vi "StateNoteHandling.vi"(0 "Master State In":T1(ring)) -> ()   [LabVIEW 2023]
doc: "This VI performs all of the calculations and decisions related to the swerve drive."
uses:
  <vilib>/Rock Robotics/WPI/ThirdParty/REV Robotics/REVLib/Typedef/Spark MAX Limit Switch Polarity.ctl
  5f0eb4dc-af05-48a2-bc5f-2393b2339903.vi
  GlobalDriverStationCommands.vi
  GlobalElevator.vi
  GlobalNoteHandling.vi
  GlobalPoseAndTargeting.vi
  GlobalShooter.vi
  GlobalDriverStationData.vi
panel:
  in  "Intake Outake Power":dbl=0.4
  in  "Outer Roller Outake Power":dbl=-0.3
  in  "Indexer Shooting Power":dbl=0.4
  in  "Indexer Reverse Power":dbl=0.1
  in  "Roller Heading Threshold":u32=10000
  in  "Outer Roller Power":dbl=0.4
  in  "Indexer Power":dbl=0.6
  in  "Intake Power":dbl=-0.4
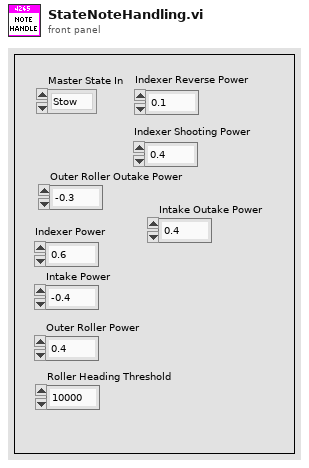
[diagram p1: front panel]
types:
  T1 = enum16{"Stow", "Speaker", "Amp", "Climbing", "Trap"}
  T2 = typedef "WPI_MotorControlDeviceRef.ctl" = cluster{"DeviceStatus":errorcluster, "Type":T3, "PWM":cluster{"PWM Channel":T4, "DeadBand":T5}, "CAN":cluster{"Device Number":u8, "SetOutput VI Ref":variant, "GetOutput VI Ref":variant, "Enable VI Ref":variant, "Disable VI Ref":variant, "Data":variant}, "Invert":bool, "DIO PWM":cluster{"PWM \"Enable\" Channel":T4, "DIOChannel":T6, "PWM Rate":dbl}}
  T3 = typedef "WPI_MotorControlType.ctl" = enum16{"PWM", "CAN", "DIO PWM"}
  T4 = typedef "FPGA_DIOPWMChannel.ctl" = enum8{"PWM 0", "PWM 1", "PWM 2", "PWM 3", "PWM 4", "PWM 5", "PWM 6", "PWM 7", "PWM 8", "PWM 9", "PWM MXP 0", "PWM MXP 1", "PWM MXP 2", "PWM MXP 3", "PWM MXP 4", "PWM MXP 5", "PWM MXP 6", "PWM MXP 7", "PWM MXP 8", "PWM MXP 9", "Invalid"}
  T5 = typedef "WPI_PWMDeadband.ctl" = cluster{"Name":string, "maxPositivePwm":i32, "minPositivePwm":i32, "centerPwm":i32, "maxNegativePwm":i32, "minNegativePwm":i32, "angularRange":u16}
  T6 = typedef "FPGA_DIOChannel.ctl" = enum8{"DIO 0", "DIO 1", "DIO 2", "DIO 3", "DIO 4", "DIO 5", "DIO 6", "DIO 7", "DIO 8", "DIO 9", "DIO MXP 0", "DIO MXP 1", "DIO MXP 2", "DIO MXP 3", "DIO MXP 4", "DIO MXP 5", "DIO MXP 6", "DIO MXP 7", "DIO MXP 8", "DIO MXP 9", "DIO MXP 10", "DIO MXP 11", "DIO MXP 12", "DIO MXP 13", "DIO MXP 14", "DIO MXP 15", "SPI Port CS1", "SPI Port CS2", "SPI Port CS3", "SPI Port MISO", "SPI Port MOSI", "Invalid"}
  T7 = typedef "Spark MAX Limit Switch Polarity.ctl" = enum16{"Normally Open", "Normally Closed"}
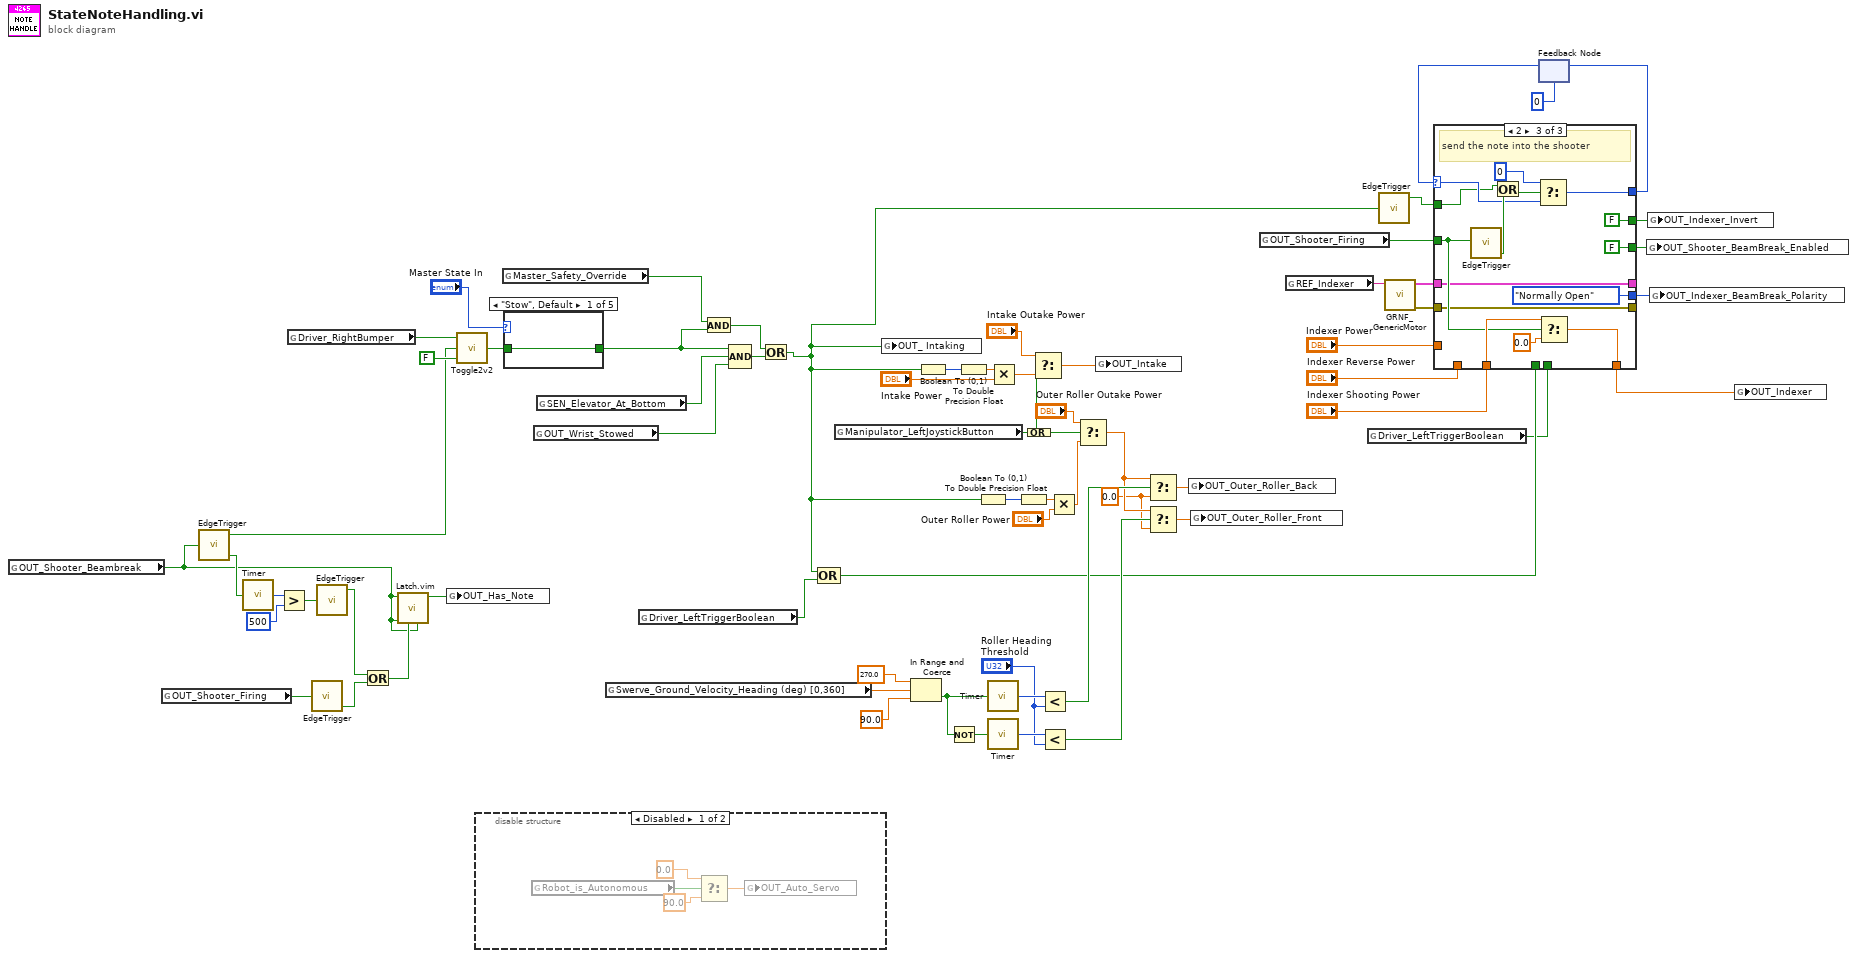
[diagram p0: block diagram]
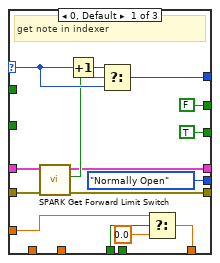
[diagram p3: hidden frame]
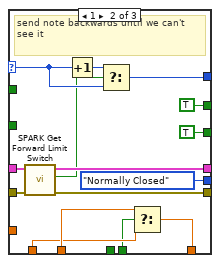
[diagram p4: hidden frame]
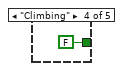
[diagram p7: hidden frame]
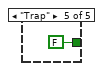
[diagram p8: hidden frame]
diagram:
  w47 = 0.0 ("f")
  n1 = global read "GlobalNoteHandling.vi" "OUT_Shooter_Beambreak"() -> (w10:bool)
  n2 = global read "GlobalShooter.vi" "OUT_Shooter_Firing"() -> (w15:bool)
  n3 = call "EdgeTrigger.vi"("Input Signal"=w10) -> ("Rising Edge Trigger"=w27:bool, "Falling Edge Trigger"=w11:bool)  [unwired: 1 out]
  n4 = call "Timer.vi"("Reset Timer"=w11) -> ("Time (ms)"=w9:u32)
  n5 = Greater?(x=w9, y=u32 500) -> (0:w7:bool)
  n6 = global read "GlobalDriverStationCommands.vi" "Driver_RightBumper"() -> (w30:bool)
  n7 = call "EdgeTrigger.vi"("Input Signal"=w15) -> ("Falling Edge Trigger"=w12:bool)  [unwired: 2 out]
  n8 = call "EdgeTrigger.vi"("Input Signal"=w7) -> ("Rising Edge Trigger"=w6:bool)  [unwired: 2 out]
  n9 = Or(x=w6, y=w12) -> (x .or. y?=w14:bool)
  n10 = call "Latch.vim"("Default Value"=w10, "Reset"=w14, "Latch Signal"=w10, "Latch Value"=w10) -> ("Latched"=w13:bool)  [unwired: 7 in]
  n11 = global write "GlobalNoteHandling.vi" "OUT_Has_Note"(w13) -> ()
  n12 = call "Toggle2v2.vi"("Initial State"=FALSE, "Reset"=w27, "Trigger"=w30) -> ("New State"=w29:bool)
  n13 = disable-structure shown="Disabled" {
    frame Disabled {
      n14 = global read "GlobalDriverStationData.vi" "Robot_is_Autonomous"() -> (w71:bool)
      n15 = Select(t=0.0, s=w71, f=90.0) -> (s? t:f=w68:dbl)
      n16 = global write "GlobalNoteHandling.vi" "OUT_Auto_Servo"(w68) -> ()
    }
    frame Enabled {
    }
  }
  n17 = global read "GlobalDriverStationData.vi" "Master_Safety_Override"() -> (w2:bool)
  n18 = case shown="\"Stow\", Default" "Master State In" {
    tunnel: w29 -> [w72 w73 w74 _ _]
    tunnel: [w72 w73 w74 FALSE FALSE] -> w3
    frame "Stow", Default {
    }
    frame "Speaker" {
    }
    frame "Amp" {
    }
    frame "Climbing" {
    }
    frame "Trap" {
    }
  }
  n19 = global read "GlobalShooter.vi" "OUT_Wrist_Stowed"() -> (w44:bool)
  n20 = global read "GlobalElevator.vi" "SEN_Elevator_At_Bottom"() -> (w59:bool)
  n21 = global read "GlobalPoseAndTargeting.vi" "Swerve_Ground_Velocity_Heading (deg) [0,360]"() -> (w58:dbl)
  n22 = global read "GlobalDriverStationCommands.vi" "Driver_LeftTriggerBoolean"() -> (w60:bool)
  n23 = And(x=w2, y=w3) -> (x .and. y?=w1:bool)
  n24 = Compound Arithmetic op=AND(w3, w59, w44) -> (w5:bool)
  n25 = Or(x=w1, y=w5) -> (x .or. y?=w4:bool)
  n26 = Compound Arithmetic op=OR(w4, w60) -> (w40:bool)
  n27 = global read "GlobalDriverStationCommands.vi" "Manipulator_LeftJoystickButton"() -> (w22:bool)
  n28 = global write "GlobalNoteHandling.vi" "OUT_ Intaking"(w4) -> ()
  n29 = In Range and Coerce(upper limit=270.0, x=w58, lower limit=90.0) -> (In Range?=w55:bool)  [unwired: 1 out]
  n30 = Boolean To (0,1)(Boolean=w4) -> (0, 1=w67:i16)
  n31 = Not(x=w55) -> (.not. x?=w54:bool)
  n32 = To Double Precision Float(number=w67) -> (double precision float=w65:dbl)
  n33 = Boolean To (0,1)(Boolean=w4) -> (0, 1=w64:i16)
  n34 = call "Timer.vi"("Reset Timer"=w55) -> ("Time (ms)"=w53:u32)
  n35 = call "Timer.vi"("Reset Timer"=w54) -> ("Time (ms)"=w52:u32)
  n36 = Multiply(x=w65, y="Intake Power") -> (x*y=w23:dbl)
  n37 = To Double Precision Float(number=w64) -> (double precision float=w63:dbl)
  n38 = Compound Arithmetic op=OR(w22) -> (w25:bool)
  n39 = Select(t="Intake Outake Power", s=w22, f=w23) -> (s? t:f=w20:dbl)
  n40 = Less?(x=w53, y="Roller Heading Threshold") -> (x < y?=w50:bool)
  n41 = Less?(x=w52, y="Roller Heading Threshold") -> (x < y?=w49:bool)
  n42 = Multiply(x=w63, y="Outer Roller Power") -> (x*y=w62:dbl)
  n43 = Select(t="Outer Roller Outake Power", s=w25, f=w62) -> (s? t:f=w48:dbl)
  n44 = global write "GlobalNoteHandling.vi" "OUT_Intake"(w20) -> ()
  n45 = Select(t=w48, s=w50, f=w47) -> (s? t:f=w45:dbl)
  n46 = Select(t=w48, s=w49, f=w47) -> (s? t:f=w46:dbl)
  n47 = global write "GlobalNoteHandling.vi" "OUT_Outer_Roller_Back"(w45) -> ()
  n48 = global write "GlobalNoteHandling.vi" "OUT_Outer_Roller_Front"(w46) -> ()
  n49 = global read "GlobalShooter.vi" "OUT_Shooter_Firing"() -> (w17:bool)
  n50 = global read "GlobalNoteHandling.vi" "REF_Indexer"() -> (w34:string)
  n51 = global read "GlobalDriverStationCommands.vi" "Driver_LeftTriggerBoolean"() -> (w24:bool)
  n52 = call "EdgeTrigger.vi"("Input Signal"=w4) -> ("Rising Edge Trigger"=w16:bool)  [unwired: 2 out]
  n53 = call "GRNF_GenericMotor.vi"("RefNum Name"=w34) -> ("Error"=w35:errorcluster, "Device Reference"=w36:T2)  [unwired: 5 in]
  n54 = feedback #1(0) -> (w41:i32)
  n55 = case shown="2" w41 {
    selector: w41 -> [w87 w93 w109]
    tunnel: [Spark_MAX_Limit_Switch_Polarity."Normally Open" ("Polarity (Normally Open)") Spark_MAX_Limit_Switch_Polarity."Normally Closed" ("Polarity (Normally Open)") Spark_MAX_Limit_Switch_Polarity."Normally Open" ("Polarity (Normally Open)")] -> w32
    tunnel: [TRUE TRUE FALSE] -> w19
    tunnel: [w88 w104 w119] -> w43
    tunnel: w35 -> [w86 w102 w111]
    tunnel: w36 -> [w85 w101 w112]
    tunnel: [w83 w100 w112] -> _
    tunnel: [w82 w99 w111] -> _
    tunnel: [FALSE TRUE FALSE] -> w33
    tunnel: w40 -> [w80 _ _]
    tunnel: "Indexer Power" -> [w79 _ _]
    tunnel: [w77 w97 w115] -> w18
    tunnel: "Indexer Reverse Power" -> [_ w96 _]
    tunnel: w17 -> [_ _ w114]
    tunnel: "Indexer Shooting Power" -> [_ w98 w117]
    tunnel: w24 -> [_ w95 _]
    tunnel: w16 -> [_ _ w107]
    frame 0, Default {
      # "get note in indexer"
      n56 = call <vilib>:"SPARK Get Forward Limit Switch.vi"("error in (no error)"=w86, "MotorControlDevRef in"=w85) -> ("error out"=w82:errorcluster, "Hard Limit Fwd"=w84:bool, "MotorControlDevRef out"=w83:T2)  [unwired: 6 in, 1 out]
      n57 = Increment(x=w87) -> (x+1=w89:i32)
      n58 = Select(t=w89, s=w84, f=w87) -> (s? t:f=w88:i32)
      n59 = Select(t=w79, s=w80, f=0.0) -> (s? t:f=w77:dbl)
    }
    frame 1 {
      # "send note backwards until we can't see it"
      n60 = call <vilib>:"SPARK Get Forward Limit Switch.vi"("error in (no error)"=w102, "MotorControlDevRef in"=w101) -> ("error out"=w99:errorcluster, "Hard Limit Fwd"=w92:bool, "MotorControlDevRef out"=w100:T2)  [unwired: 6 in, 1 out]
      n61 = Increment(x=w93) -> (x+1=w94:i32)
      n62 = Select(t=w94, s=w92, f=w93) -> (s? t:f=w104:i32)
      n63 = Select(t=w98, s=w95, f=w96) -> (s? t:f=w97:dbl)
    }
    frame 2 {
      # "send the note into the shooter"
      n64 = call "EdgeTrigger.vi"("Input Signal"=w114) -> ("Falling Edge Trigger"=w113:bool)  [unwired: 2 out]
      n65 = Or(x=w107, y=w113) -> (x .or. y?=w108:bool)
      n66 = Select(t=0, s=w108, f=w109) -> (s? t:f=w119:i32)
      n67 = Select(t=w117, s=w114, f=0.0) -> (s? t:f=w115:dbl)
    }
  }
  n68 = feedback-in #1(w43) -> ()
  n69 = global write "GlobalNoteHandling.vi" "OUT_Shooter_BeamBreak_Enabled"(w19) -> ()
  n70 = global write "GlobalNoteHandling.vi" "OUT_Indexer_Invert"(w33) -> ()
  n71 = global write "GlobalNoteHandling.vi" "OUT_Indexer_BeamBreak_Polarity"(w32) -> ()
  n72 = global write "GlobalNoteHandling.vi" "OUT_Indexer"(w18) -> ()
